vi "Configure Limit Test.vi"(0 "VISA resource name":refnum<visa-resource-name>, 1 "Autoclear IO Port (T: Enable)":bool=TRUE, 5 "Limit Test Data Feed (0: Input Signal)":u16(ring) items=["Input Signal", "Math Result"], 7 "Limit Test Pass Bit Pattern (15)":u16=15, 11 "error in (no error)":errorcluster, 12 "Limit Test Line 4 Mode (0: End of Test)":u16(ring) items=["End of Test", "Busy"], 13 "Limit Test Line 4 Busy Level (0: Low)":u16(ring) items=["Low", "High"]) -> (4 "VISA resource name out":refnum<visa-resource-name>, 15 "error out":errorcluster)   [LabVIEW 2020, in "Keithley 648X Series.lvlib"]
doc: "Configures general limit test features.\n\n<b>Note:</b>\nThis VI is part of the component handler interfacing VIs."
uses:
  <instrlib>/Keithley 648X Series/Keithley 648X Series.lvlib
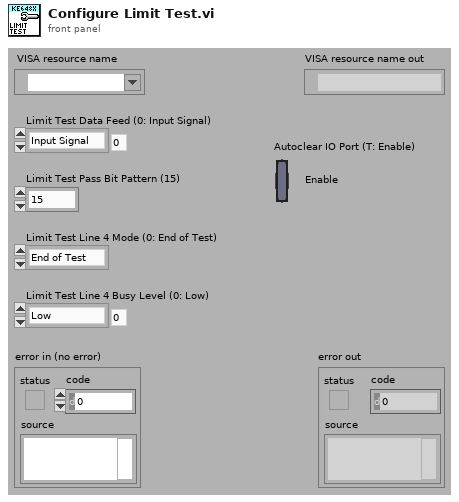
[diagram p1: front panel]
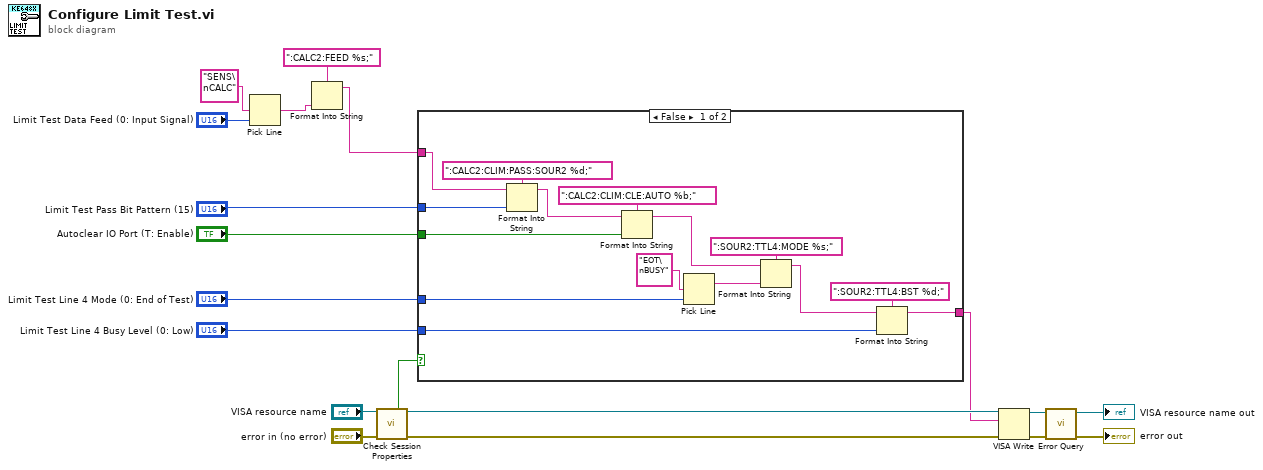
[diagram p0: block diagram]
diagram:
  n1 = Pick Line(multi-line string="SENS\nCALC", line index="Limit Test Data Feed (0: Input Signal)") -> (output string=w12:string)  [unwired: 1 in]
  n2 = Format Into String(format string=":CALC2:FEED %s;", w12) -> (resulting string=w6:string)  [unwired: 2 in, 1 out]
  n3 = call <instrlib>:"Check Session Properties.vi"("VISA resource name"="VISA resource name", "error in (no error)"="error in (no error)") -> ("Model 6485"=w7:bool, "VISA resource name out"=w11:refnum<visa-resource-name>, "error out"=w8:errorcluster)  [unwired: 10 in, 1 out]
  n4 = case shown="False" w7 {
    tunnel: w6 -> [w32 w35]
    tunnel: [w20 w35] -> w5
    tunnel: "Limit Test Pass Bit Pattern (15)" -> [w33 _]
    tunnel: "Autoclear IO Port (T: Enable)" -> [w29 _]
    tunnel: "Limit Test Line 4 Mode (0: End of Test)" -> [w26 _]
    tunnel: "Limit Test Line 4 Busy Level (0: Low)" -> [w22 _]
    frame False {
      n5 = Format Into String(format string=":CALC2:CLIM:PASS:SOUR2 %d;", initial string=w32, w33) -> (resulting string=w31:string)  [unwired: 1 in, 1 out]
      n6 = Format Into String(format string=":CALC2:CLIM:CLE:AUTO %b;", initial string=w31, w29) -> (resulting string=w24:string)  [unwired: 1 in, 1 out]
      n7 = Pick Line(multi-line string="EOT\nBUSY", line index=w26) -> (output string=w25:string)  [unwired: 1 in]
      n8 = Format Into String(format string=":SOUR2:TTL4:MODE %s;", initial string=w24, w25) -> (resulting string=w21:string)  [unwired: 1 in, 1 out]
      n9 = Format Into String(format string=":SOUR2:TTL4:BST %d;", initial string=w21, w22) -> (resulting string=w20:string)  [unwired: 1 in, 1 out]
    }
    frame True {
      # "Model 6485 doesn't have digital output operations"
    }
  }
  n10 = VISA Write(VISA resource name=w11, write buffer=w5, error in (no error)=w8) -> (VISA resource name out=w17:refnum<visa-resource-name>, error out=w16:errorcluster)  [unwired: 1 out]
  n11 = call <instrlib>:"Error Query.vi"("error in (no error)"=w16, "VISA resource name"=w17) -> ("error out"=→"error out":errorcluster, "VISA resource name out"=→"VISA resource name out":refnum<visa-resource-name>)  [unwired: 6 in, 2 out]
